vi "N4_201_write_mode.vi"(4 "Driver Name":T10, 6 "Error Code":T11, 7 "Command":T8, 8 "error in":T9, 11 "DriverConnect in":T1={"InterfaceType"=enum."VISA", "OpenedSession"="", "InterfaceSettings"={"Interface"=enum."RS232", "EOS 4 read"=enum."LF (\\n)", "EOS 4 write"=enum."LF (\\n)", "TMO, ms"=10000, "Sett"=variant(cluster{"Baud Rate":u32, "Data Bits":u16, "Parity":u16, "Stop Bits":u16, "Flow Control":u16, "Eho":bool} {"Baud Rate"=75, "Data Bits"=0, "Parity"=0, "Stop Bits"=0, "Flow Control"=0, "Eho"=FALSE})}}) -> (0 "error out":T9, 3 "DriverConnect out":T1={"InterfaceType"=enum."VISA", "OpenedSession"="", "InterfaceSettings"={"Interface"=enum."RS232", "EOS 4 read"=enum."LF (\\n)", "EOS 4 write"=enum."LF (\\n)", "TMO, ms"=10000, "Sett"=variant(cluster{"Baud Rate":u32, "Data Bits":u16, "Parity":u16, "Stop Bits":u16, "Flow Control":u16, "Eho":bool} {"Baud Rate"=75, "Data Bits"=0, "Parity"=0, "Stop Bits"=0, "Flow Control"=0, "Eho"=FALSE})}}, 5 "ModeWasChacged":T6)   [LabVIEW 2018]
uses:
  MOKO_LabViewLibrary/MokoLowLevel/MokoLowLovelControl/MLLC_ErrorCode.ctl
  MOKO_LabViewLibrary/MokoLowLevel/MokoLowLovelControl/MLLC_DriverName.ctl
  MOKO_LabViewLibrary/MokoLowLevel/MokoLowLovelControl/MLLC_Error.ctl
  MOKO_LabViewLibrary/MokoLowLevel/MokoLowLovelControl/MLLC_Command.ctl
  MOKO_LabViewLibrary/MokoLowLevel/MokoLowLovelControl/MLLC_Delay.ctl
  MOKO_LabViewLibrary/MokoLowLevel/MokoLowLovelControl/MLLC_Boolean.ctl
  MOKO_LabViewLibrary/MokoLowLevel/MokoLowLovelControl/MLLC_ConnectCluster.ctl
  MOKO_LabViewLibrary/MokoLowLevel/MokoLowLovelControl/MLLC_InterfaceType.ctl
  MOKO_LabViewLibrary/MokoLowLevel/MokoLowLovelControl/MLLC_OpenedSession.ctl
  MOKO_LabViewLibrary/MokoLowLevel/MokoLowLovelControl/MLLC_InterfaceSettings.ctl
  MOKO_LabViewLibrary/MokoLowLevel/MokoLowLovelControl/MLLC_InterfaceKind.ctl
panel:
  in  "Delay Time (s)":T7=3.0
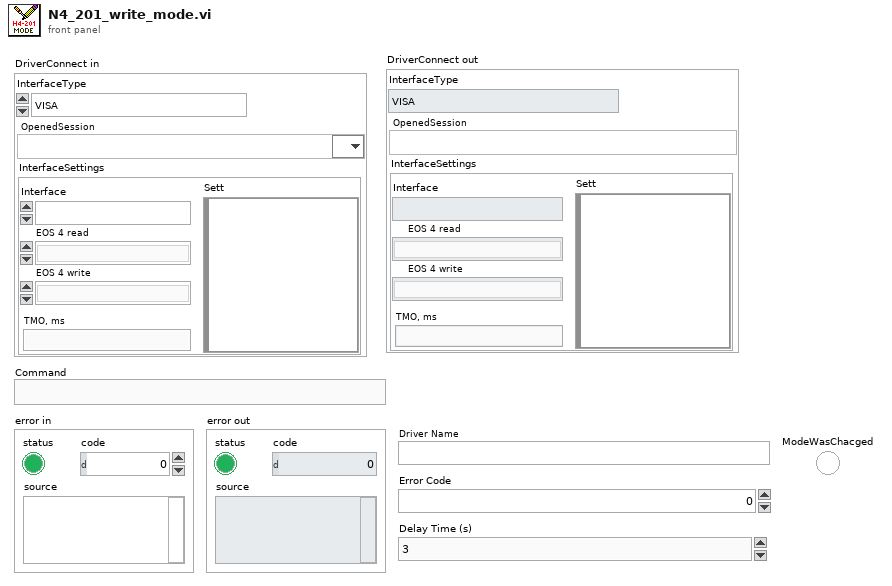
[diagram p1: front panel]
types:
  T1 = typedef "MLLC_ConnectCluster.ctl" = cluster{"InterfaceType":T2, "OpenedSession":T3, "InterfaceSettings":T4}
  T2 = typedef "MLLC_InterfaceType.ctl" = enum16{"VISA", "Prologix USB-GPIB"}
  T3 = typedef "MLLC_OpenedSession.ctl" = refnum<visa-resource-name>
  T4 = typedef "MLLC_InterfaceSettings.ctl" = cluster{"Interface":T5, "EOS 4 read":enum16{"Default (=EOS 4 write)", "CR (\\r)", "LF (\\n)", "None"}, "EOS 4 write":enum16{"CR+LF (\\r\\n)", "CR (\\r)", "LF (\\n)", "None"}, "TMO, ms":i32, "Sett":variant}
  T5 = typedef "MLLC_InterfaceKind.ctl" = enum16{"RS232", "GPIB", "USB", "Ethernet", "another"}
  T6 = typedef "MLLC_Boolean.ctl" = bool
  T7 = typedef "MLLC_Delay.ctl" = dbl
  T8 = typedef "MLLC_Command.ctl" = string
  T9 = typedef "MLLC_Error.ctl" = errorcluster
  T10 = typedef "MLLC_DriverName.ctl" = string
  T11 = typedef "MLLC_ErrorCode.ctl" = u32
  T12 = enum16{"Нет симуляции", "В ручную", "Игнорировать"}
  T13 = typedef "MLLC_Response.ctl" = string
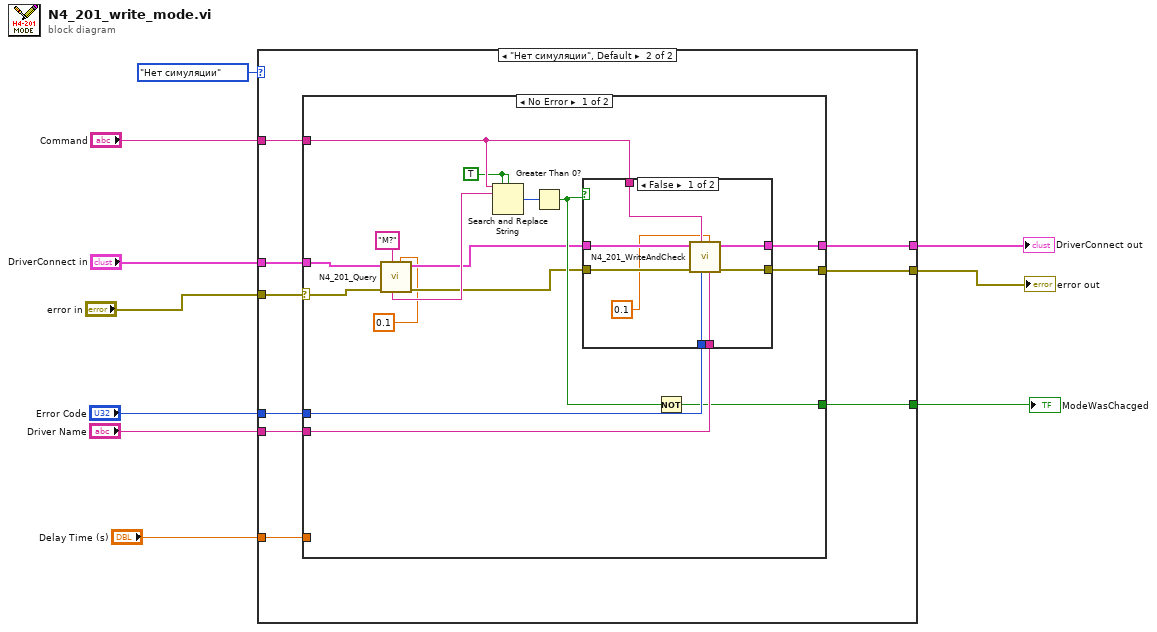
[diagram p0: block diagram]
diagram:
  n1 = case shown="\"Нет симуляции\", Default" T12."Нет симуляции" ("Simmulation") {
    tunnel: [w11 w21] -> w10
    tunnel: "Error Code" -> [_ w20]
    tunnel: "Driver Name" -> [_ w19]
    tunnel: "DriverConnect in" -> [w12 w18]
    tunnel: "error in" -> [w11 w17]
    tunnel: "Command" -> [_ w16]
    tunnel: "Delay Time (s)" -> [_ w15]
    tunnel: [w12 w14] -> w1
    tunnel: [_ w13] -> w4
    frame "В ручную" {
    }
    frame "Нет симуляции", Default {
      n2 = case shown="No Error" w17 {
        selector: w17 -> [w31 w49]
        tunnel: [w34 w49] -> w21
        tunnel: [w35 w48] -> w14
        tunnel: w20 -> [w37 _]
        tunnel: w19 -> [w36 _]
        tunnel: w18 -> [w32 w48]
        tunnel: w16 -> [w30 _]
        tunnel: w15 -> [_ _]
        tunnel: [w27 _] -> w13
        frame No Error {
          w29 = TRUE ("replace all? (F)")
          n3 = call "N4_201_Query.vi"("Delay Befor (s)"=0.1 ("Command Time (s)"), "Command"="M?" ("Error Query"), "error in"=w31, "DriverConnect in"=w32) -> ("error out"=w23:T9, "DriverConnect out"=w24:T1, "Response"=w25:T13)  [unwired: 5 in]
          n4 = Search and Replace String(replace all?=w29, case sensitive?=w29, input string=w30, search string=w25) -> (number of replacements=w28:i32)  [unwired: 4 in, 3 out]
          n5 = Greater Than 0?(x=w28) -> (x > 0?=w26:bool)
          n6 = case shown="False" w26 {
            tunnel: w37 -> [w45 _]
            tunnel: w36 -> [w44 _]
            tunnel: [w43 w47] -> w35
            tunnel: [w39 w46] -> w34
            tunnel: w30 -> [w42 _]
            tunnel: w24 -> [w41 w47]
            tunnel: w23 -> [w40 w46]
            frame False {
              n7 = call "N4_201_WriteAndCheck.vi"("Driver Name"=w44, "Command Time (s)"=0.1, "Error Code"=w45, "Command"=w42, "error in"=w40, "DriverConnect in"=w41) -> ("error out"=w39:T9, "DriverConnect out"=w43:T1)  [unwired: 4 in]
            }
            frame True {
            }
          }
          n8 = Not(x=w26) -> (.not. x?=w27:bool)
        }
        frame Error {
        }
      }
    }
  }
  "error out" <- w10
  "ModeWasChacged" <- w4
  "DriverConnect out" <- w1
